vi "encoder_display.vi"() -> ()   [LabVIEW 2011]
panel:
  out "Velocidad del Motor":dbl(graph)
  in  "Vout":dbl(slide) scale=-10.0..10.0
  in  "VISA COM IN":refnum<visa-resource-name>
  in  "stop":bool
  # "Velocidad del Motor"
  # "Voltaje de salida"
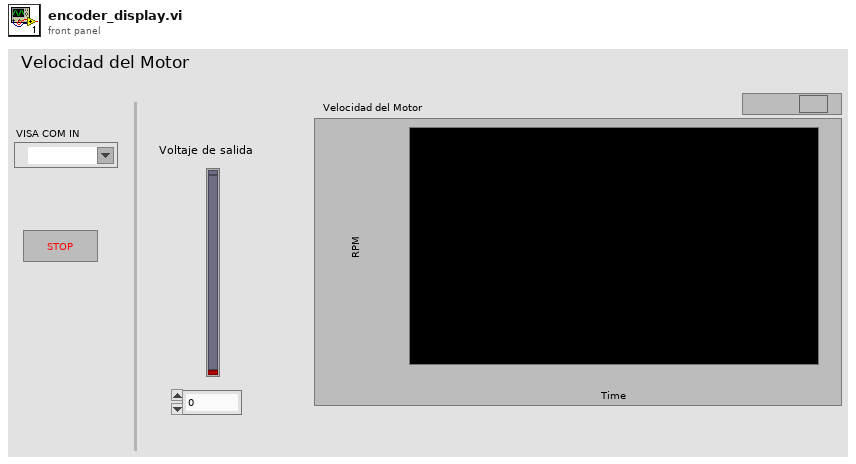
[diagram p1: front panel]
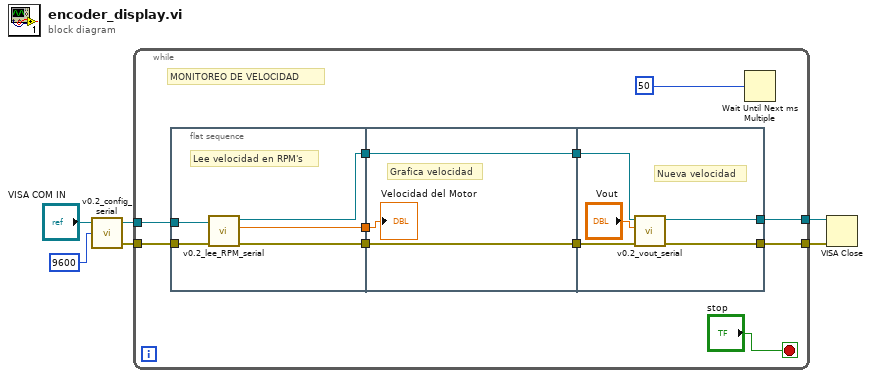
[diagram p0: block diagram]
diagram:
  n1 = call "v0.2_config_serial.vi"("baud rate (9600/115200)"=u32 9600, "VISA COM IN"="VISA COM IN") -> ("error out"=w3:errorcluster, "VISA COM OUT"=w4:refnum<visa-resource-name>)  [unwired: 2 in]
  n2 = while {
    tunnel: w4 -> [w15]
    tunnel: w3 -> [w14]
    tunnel: [w8] -> w2
    tunnel: [w7] -> w1
    stop <- "stop" stop-if-true
    # "MONITOREO DE VELOCIDAD"
    n3 = flat-sequence {
      tunnel: w15 -> [w22]
      tunnel: w14 -> [w21]
      tunnel: [w20] -> w13
      tunnel: [w19] -> w11
      tunnel: [w18] -> w9
      tunnel: w13 -> [w25]
      tunnel: [w24] -> w12
      tunnel: w11 -> [w24]
      tunnel: [w23] -> w10
      tunnel: w9 -> [w23]
      tunnel: w12 -> [w29]
      tunnel: w10 -> [w28]
      tunnel: [w27] -> w8
      tunnel: [w26] -> w7
      frame #0 {
        # "Lee velocidad en RPM's"
        n4 = call "v0.2_lee_RPM_serial.vi"("error in (no error)"=w21, "VISA COM IN"=w22) -> ("error out"=w18:errorcluster, "RPM"=w20:dbl, "VISA COM OUT"=w19:refnum<visa-resource-name>)  [unwired: 7 in]
      }
      frame #1 {
        # "Grafica velocidad"
        "Velocidad del Motor" <- w25
      }
      frame #2 {
        # "Nueva velocidad"
        n5 = call "v0.2_vout_serial.vi"("error in (no error)"=w28, "Volt"="Vout", "VISA COM IN"=w29) -> ("error out"=w26:errorcluster, "VISA COM OUT"=w27:refnum<visa-resource-name>)  [unwired: 7 in]
      }
    }
    n6 = Wait Until Next ms Multiple(millisecond multiple=u32 50) -> ()  [unwired: 1 out]
  }
  n7 = VISA Close(VISA resource name=w2, error in (no error)=w1) -> ()  [unwired: 1 out]
